vi "Setcondition.vi"(8 "error in (no error)":errorcluster, 10 "Set_Val":T1, 11 "OneOfTemplate in":refnum<class "nixnet_grpc_WaitRequest_condition_enum.lvclass">) -> (0 "error out":errorcluster, 3 "OneOfTemplate out":refnum<class "nixnet_grpc_WaitRequest_condition_enum.lvclass">)   [LabVIEW 2019, in "xnet-grpc_client.lvlib" / "nixnet_grpc_WaitRequest_condition_enum.lvclass"]
uses:
  nixnet_grpc_WaitRequest_condition_enum.lvclass
  nixnet_grpc_WaitCondition.ctl
  nixnet_grpc_WaitRequest_condition_enum.lvclass/nixnet_grpc_WaitRequest_condition_enum.ctl
  xnet-grpc_client.lvlib
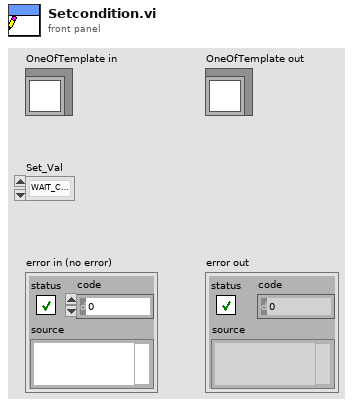
[diagram p1: front panel]
types:
  T1 = typedef "xnet-grpc_client.lvlib/nixnet_grpc_WaitCondition.ctl" = enum32{"WAIT_CONDITION_UNSPECIFIED", "WAIT_CONDITION_TRANSMIT_COMPLETE", "WAIT_CONDITION_INTF_COMMUNICATING", "WAIT_CONDITION_INTF_REMOTE_WAKEUP", "WAIT_CONDITION_ETHERNET_SYNCED"}
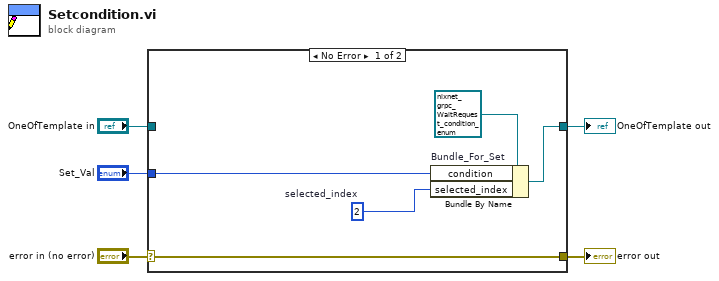
[diagram p0: block diagram]
diagram:
  n1 = case shown="No Error" "error in (no error)" {
    selector: "error in (no error)" -> [w10 w11]
    tunnel: [w10 w11] -> w4
    tunnel: [w9 w12] -> w2
    tunnel: "OneOfTemplate in" -> [_ w12]
    tunnel: "Set_Val" -> [w8 _]
    frame No Error {
      w7 = 2  # selected_index
      n2 = Bundle By Name "Bundle_For_Set"(cluster=refnum<class "nixnet_grpc_WaitRequest_condition_enum.lvclass"> refnum ("OneOfTemplate in"), "condition"=w8, "selected_index"=w7) -> (w9:refnum<class "nixnet_grpc_WaitRequest_condition_enum.lvclass">)
    }
    frame Error {
    }
  }
  "error out" <- w4
  "OneOfTemplate out" <- w2
